vi "Get Base Paths.vi"() -> (2 "Stimulus Profiles Logging Base Path Folder Out":path, 3 "Stimulus Profiles Base Path Folder Out":path)   [LabVIEW 2010]
doc: "This VI requires a user to input a path folder for the stimulus profiles and where they want the stimulus profile logs to be stored."
panel:
  in  "Stimulus Profiles Logging Base Path Folder":path
  in  "DONE":bool
  in  "Stimulus Profiles Base Path Folder":path
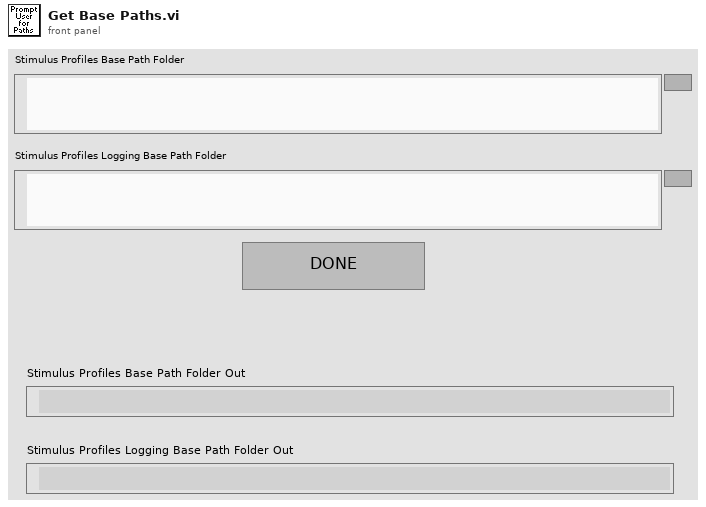
[diagram p1: front panel]
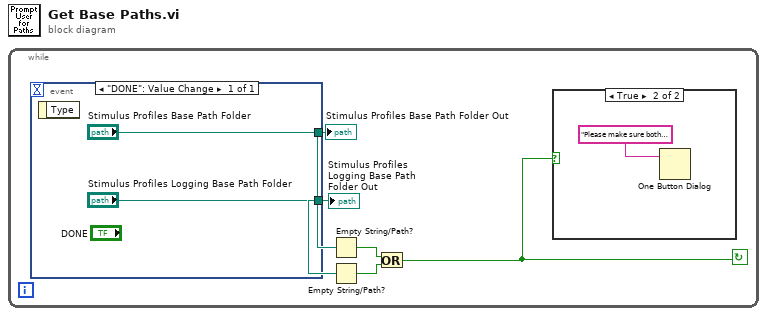
[diagram p0: block diagram]
diagram:
  n1 = while {
    stop <- w1 continue-if-true
    n2 = event shown="[0] \"DONE\": Value Change" {
      selector: _ -> [_]
      dyn-events: _ -> [_]
      timeout: _ -> [_]
      tunnel: ["Stimulus Profiles Base Path Folder"] -> w3
      tunnel: ["Stimulus Profiles Logging Base Path Folder"] -> w2
      event "DONE": Value Change {
        n3 = event-data() -> ()  [unwired: 1 in, 1 out]
      }
    }
    "Stimulus Profiles Base Path Folder Out" <- w3
    "Stimulus Profiles Logging Base Path Folder Out" <- w2
    n4 = Empty String/Path?(string/path=w3) -> (empty?=w5:bool)
    n5 = Empty String/Path?(string/path=w2) -> (empty?=w4:bool)
    n6 = Or(x=w5, y=w4) -> (x .or. y?=w1:bool)
    n7 = case shown="True" w1 {
      frame False {
      }
      frame True {
        n8 = One Button Dialog(message="Please make sure both inputs have valid folder paths") -> ()  [unwired: 1 in, 1 out]
      }
    }
  }
